vi "Packet Strings to Values.vi"(11 "Pakcet Values":string[](array[string])) -> (3 "Data Report":T1)   [LabVIEW 2013]
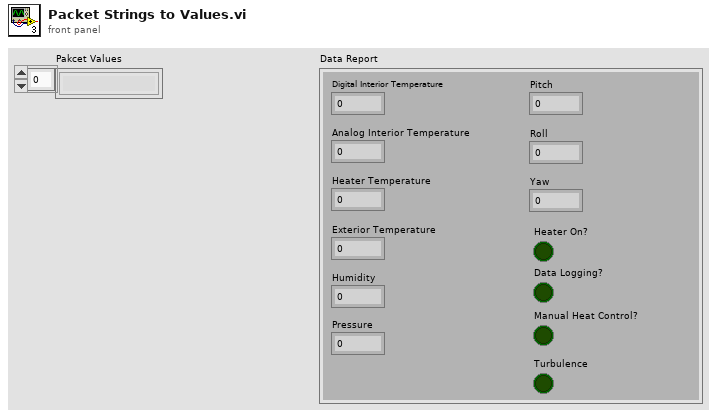
[diagram p1: front panel]
types:
  T1 = cluster{"Digital Interior Temperature":dbl, "Analog Interior Temperature":dbl, "Heater Temperature":dbl, "Exterior Temperature":dbl, "Humidity":dbl, "Pressure":dbl, "Pitch":dbl, "Roll":dbl, "Yaw":dbl, "Heater On?":bool, "Data Logging?":bool, "Manual Heat Control?":bool, "Turbulence":bool}
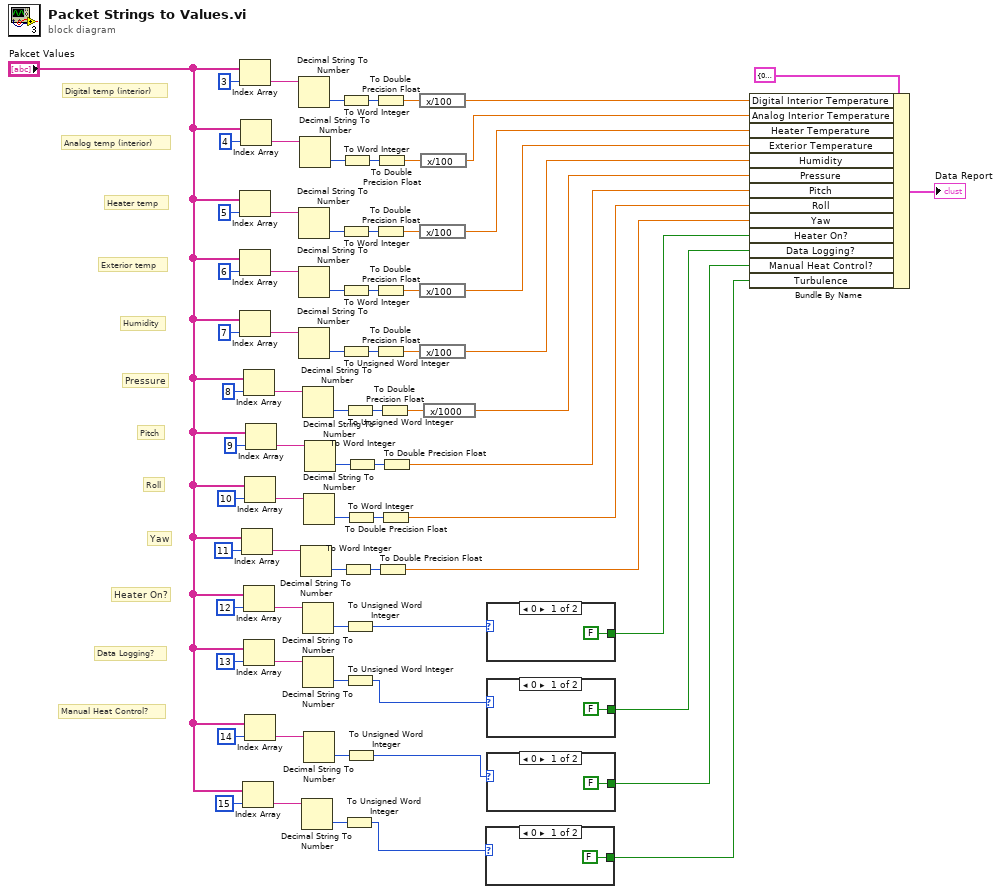
[diagram p0: block diagram]
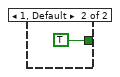
[diagram p2: hidden frame]
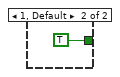
[diagram p3: hidden frame]
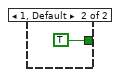
[diagram p4: hidden frame]
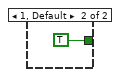
[diagram p5: hidden frame]
diagram:
  # "Manual Heat Control?"
  # "Data Logging?"
  # "Heater On?"
  # "Yaw"
  # "Roll"
  # "Pitch"
  # "Pressure"
  # "Humidity"
  # "Exterior temp"
  # "Heater temp"
  # "Analog temp (interior)"
  # "Digital temp (interior)"
  n1 = Index Array(array="Pakcet Values", index=3) -> (element=w72:string)
  n2 = Index Array(array="Pakcet Values", index=5) -> (element=w62:string)
  n3 = Index Array(array="Pakcet Values", index=6) -> (element=w57:string)
  n4 = Index Array(array="Pakcet Values", index=7) -> (element=w52:string)
  n5 = Index Array(array="Pakcet Values", index=4) -> (element=w67:string)
  n6 = Index Array(array="Pakcet Values", index=11) -> (element=w34:string)
  n7 = Index Array(array="Pakcet Values", index=15) -> (element=w4:string)
  n8 = Index Array(array="Pakcet Values", index=8) -> (element=w47:string)
  n9 = Index Array(array="Pakcet Values", index=12) -> (element=w30:string)
  n10 = Index Array(array="Pakcet Values", index=13) -> (element=w27:string)
  n11 = Index Array(array="Pakcet Values", index=10) -> (element=w38:string)
  n12 = Index Array(array="Pakcet Values", index=14) -> (element=w11:string)
  n13 = Index Array(array="Pakcet Values", index=9) -> (element=w42:string)
  n14 = Decimal String To Number(string=w72) -> (number=w73:i32)  [unwired: 2 in, 1 out]
  n15 = Decimal String To Number(string=w62) -> (number=w63:i32)  [unwired: 2 in, 1 out]
  n16 = Decimal String To Number(string=w57) -> (number=w58:i32)  [unwired: 2 in, 1 out]
  n17 = Decimal String To Number(string=w52) -> (number=w53:i32)  [unwired: 2 in, 1 out]
  n18 = Decimal String To Number(string=w67) -> (number=w68:i32)  [unwired: 2 in, 1 out]
  n19 = Decimal String To Number(string=w34) -> (number=w35:i32)  [unwired: 2 in, 1 out]
  n20 = Decimal String To Number(string=w4) -> (number=w5:i32)  [unwired: 2 in, 1 out]
  n21 = Decimal String To Number(string=w47) -> (number=w48:i32)  [unwired: 2 in, 1 out]
  n22 = Decimal String To Number(string=w30) -> (number=w31:i32)  [unwired: 2 in, 1 out]
  n23 = Decimal String To Number(string=w27) -> (number=w28:i32)  [unwired: 2 in, 1 out]
  n24 = Decimal String To Number(string=w38) -> (number=w39:i32)  [unwired: 2 in, 1 out]
  n25 = Decimal String To Number(string=w11) -> (number=w12:i32)  [unwired: 2 in, 1 out]
  n26 = Decimal String To Number(string=w42) -> (number=w43:i32)  [unwired: 2 in, 1 out]
  n27 = To Word Integer(number=w73) -> (16bit integer=w71:i16)
  n28 = To Word Integer(number=w63) -> (16bit integer=w61:i16)
  n29 = To Word Integer(number=w58) -> (16bit integer=w56:i16)
  n30 = To Unsigned Word Integer(number=w53) -> (unsigned 16bit integer=w51:u16)
  n31 = To Word Integer(number=w68) -> (16bit integer=w66:i16)
  n32 = To Word Integer(number=w35) -> (16bit integer=w33:i16)
  n33 = To Unsigned Word Integer(number=w5) -> (unsigned 16bit integer=w2:u16)
  n34 = To Unsigned Word Integer(number=w48) -> (unsigned 16bit integer=w46:u16)
  n35 = To Unsigned Word Integer(number=w31) -> (unsigned 16bit integer=w20:u16)
  n36 = To Unsigned Word Integer(number=w28) -> (unsigned 16bit integer=w18:u16)
  n37 = To Word Integer(number=w39) -> (16bit integer=w37:i16)
  n38 = To Unsigned Word Integer(number=w12) -> (unsigned 16bit integer=w10:u16)
  n39 = To Word Integer(number=w43) -> (16bit integer=w41:i16)
  n40 = To Double Precision Float(number=w71) -> (double precision float=w70:dbl)
  n41 = To Double Precision Float(number=w61) -> (double precision float=w60:dbl)
  n42 = To Double Precision Float(number=w56) -> (double precision float=w55:dbl)
  n43 = To Double Precision Float(number=w51) -> (double precision float=w50:dbl)
  n44 = To Double Precision Float(number=w66) -> (double precision float=w65:dbl)
  n45 = To Double Precision Float(number=w33) -> (double precision float=w16:dbl)
  n46 = To Double Precision Float(number=w46) -> (double precision float=w45:dbl)
  n47 = To Double Precision Float(number=w37) -> (double precision float=w15:dbl)
  n48 = To Double Precision Float(number=w41) -> (double precision float=w14:dbl)
  n49 = expression code="x/100"(w70) -> (w26:dbl)
  n50 = expression code="x/100"(w60) -> (w24:dbl)
  n51 = expression code="x/100"(w55) -> (w23:dbl)
  n52 = expression code="x/100"(w50) -> (w22:dbl)
  n53 = expression code="x/100"(w65) -> (w25:dbl)
  n54 = expression code="x/1000"(w45) -> (w21:dbl)
  n55 = case shown="0" w2 {
    tunnel: [FALSE TRUE] -> w1
    frame 0 {
    }
    frame 1, Default {
    }
  }
  n56 = case shown="0" w20 {
    tunnel: [FALSE TRUE] -> w19
    frame 0 {
    }
    frame 1, Default {
    }
  }
  n57 = case shown="0" w18 {
    tunnel: [FALSE TRUE] -> w17
    frame 0 {
    }
    frame 1, Default {
    }
  }
  n58 = case shown="0" w10 {
    tunnel: [FALSE TRUE] -> w9
    frame 0 {
    }
    frame 1, Default {
    }
  }
  n59 = Bundle By Name(cluster=T1 {"Digital Interior Temperature"=0.0, "Analog Interior Temperature"=0.0, "Heater Temperature"=0.0, "Exterior Temperature"=0.0, "Humidity"=0.0, "Pressure"=0.0, "Pitch"=0.0, "Roll"=0.0, "Yaw"=0.0, "Heater On?"=FALSE, "Data Logging?"=FALSE, "Manual Heat Control?"=FALSE, "Turbulence"=FALSE} ("Data Report"), "Digital Interior Temperature"=w26, "Analog Interior Temperature"=w25, "Heater Temperature"=w24, "Exterior Temperature"=w23, "Humidity"=w22, "Pressure"=w21, "Pitch"=w14, "Roll"=w15, "Yaw"=w16, "Heater On?"=w19, "Data Logging?"=w17, "Manual Heat Control?"=w9, "Turbulence"=w1) -> (→"Data Report":T1)
